vi "Main.vi"() -> ()   [LabVIEW 2020]
uses:
  Ctrl/Ctrl_FGV_state.ctl
panel:
  out "error out":errorcluster caption="sortie d'erreur"
  in  "error in":errorcluster caption="entrée d'erreur"
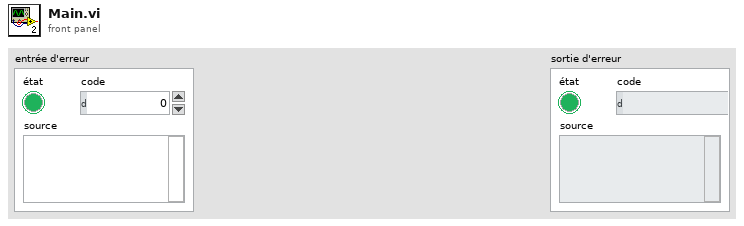
[diagram p1: front panel]
types:
  T1 = typedef "Ctrl_FGV_state.ctl" = enum16{"Init", "Read", "Write File", "Read File"}
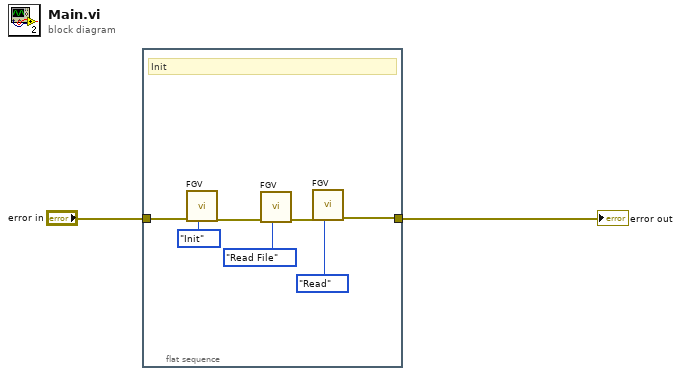
[diagram p0: block diagram]
diagram:
  n1 = flat-sequence {
    tunnel: "error in" -> [w9]
    tunnel: [w3] -> w1
    frame #0 {
      # "Init"
      n2 = call "FGV.vi"("FGV state"=Ctrl_FGV_state."Init", "error in"=w9) -> ("error out"=w7:errorcluster)  [unwired: 8 in, 1 out]
      n3 = call "FGV.vi"("FGV state"=Ctrl_FGV_state."Read File", "error in"=w7) -> ("error out"=w5:errorcluster)  [unwired: 8 in, 1 out]
      n4 = call "FGV.vi"("FGV state"=Ctrl_FGV_state."Read", "error in"=w5) -> ("error out"=w3:errorcluster)  [unwired: 8 in, 1 out]
    }
  }
  "error out" <- w1
